vi "Initialize Globals - Engineering.vi"(0 "TSM context":T2, 5 "TCs-Engineering":T1) -> (15 "error out":errorcluster)   [LabVIEW 2019]
uses:
  <vilib>/NI_TestStand_SemiconductorModule/NI_TestStand_Semiconductor_Module.lvlibp/PinMap/General/SemiconductorModuleContext.ctl
  Common/Utility/typedefs/TCs-Engineering.ctl
  TSM Context Data Access/TSM Context Data Access.lvclass/TSM Context Data Access.ctl
  TSM Context Data Access/Public/Properties/TCs-Engineering - Write.vi
  <vilib>/NI_TestStand_SemiconductorModule/NI_TestStand_Semiconductor_Module.lvlibp/PinMap/Site and Global Data/SetGlobalData.vi
  TSM Context Data Access/TSM Context Data Access.lvclass
  <vilib>/NI_TestStand_SemiconductorModule/NI_TestStand_Semiconductor_Module.lvlibp
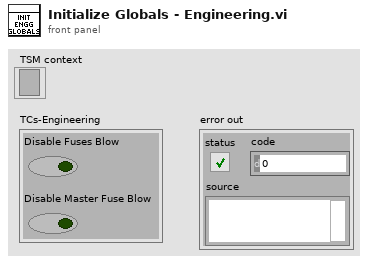
[diagram p1: front panel]
types:
  T1 = typedef "TCs-Engineering.ctl" = cluster{"Disable Fuses Blow":bool, "Disable Master Fuse Blow":bool}
  T2 = typedef "NI_TestStand_Semiconductor_Module.lvlibp/SemiconductorModuleContext.ctl" = refnum<k7>
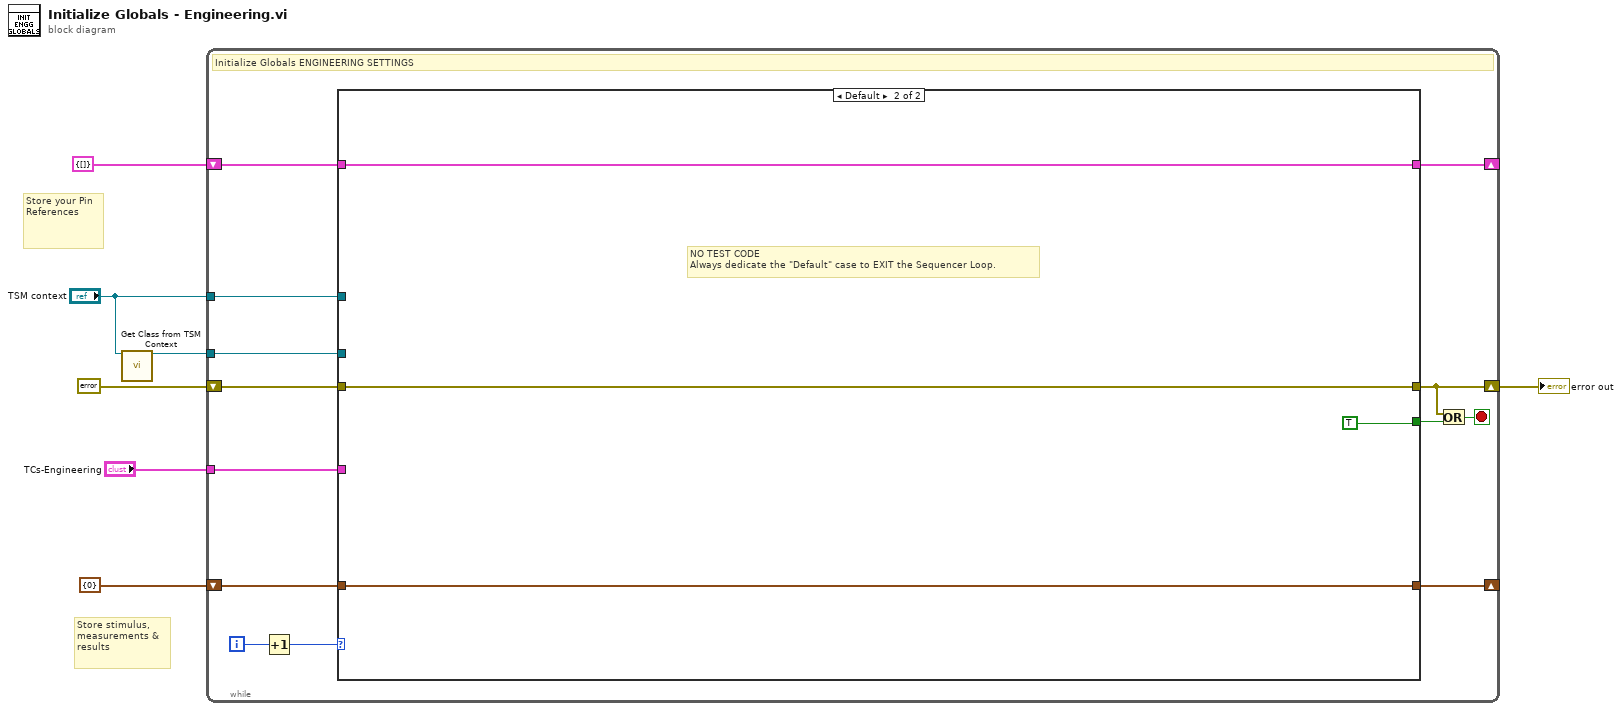
[diagram p0: block diagram]
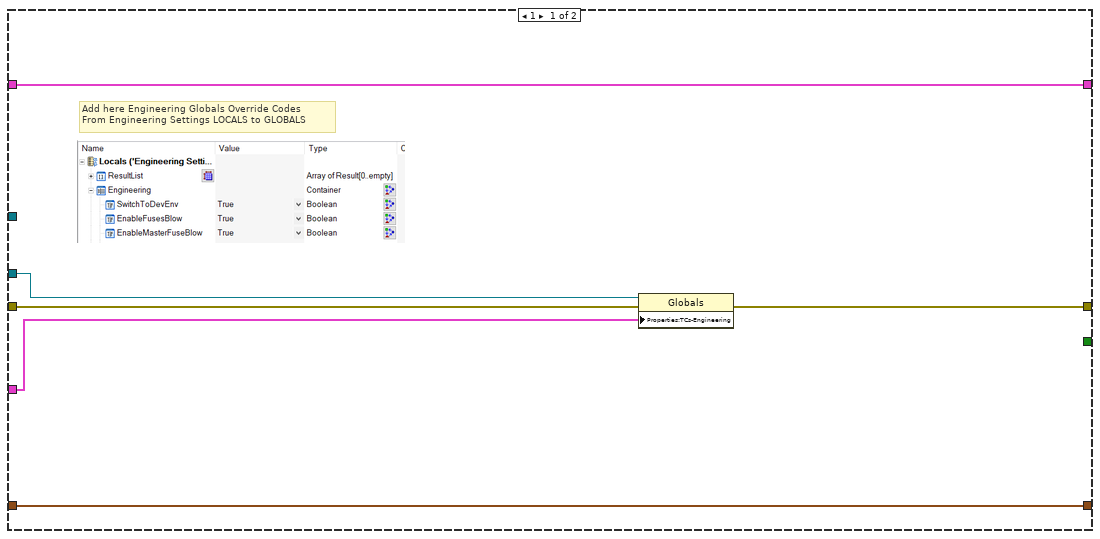
[diagram p2: hidden frame]
diagram:
  # "Store stimulus, measurements & results"
  # "Store your Pin References"
  n1 = call "Get Class from TSM Context.vi"("TSM Context"="TSM context") -> ("Global Memory Class"=w2:refnum<class "TSM Context Data Access.lvclass">)  [unwired: 14 in]
  n2 = while {
    shift-right: [w12] -> w7
    shift-left: errorcluster {"status"=FALSE, "code"=0, "source"=""} ("error in") -> [w19]
    tunnel: "TSM context" -> [w17]
    shift-right: [w14] -> _
    shift-left: cluster{"Site Numbers":i32[]} {"Site Numbers"=[]} -> [w15]
    shift-right: [w11] -> _
    shift-left: cluster{"Sample Control":i32} {"Sample Control"=0} ("TCs") -> [w10]
    tunnel: w2 -> [w9]
    tunnel: "TCs-Engineering" -> [w8]
    i -> [w20]
    stop <- w13 stop-if-true
    # "Initialize Globals ENGINEERING SETTINGS"
    n3 = Increment(x=w20) -> (x+1=w18:i32)
    n4 = case shown="Default" w18 {
      tunnel: [w23 w29] -> w12
      tunnel: w19 -> [w24 w29]
      tunnel: w17 -> [_ _]
      tunnel: [_ TRUE] -> w16
      tunnel: w15 -> [w26 w28]
      tunnel: [w26 w28] -> w14
      tunnel: [w25 w27] -> w11
      tunnel: w10 -> [w25 w27]
      tunnel: w9 -> [w22 _]
      tunnel: w8 -> [w21 _]
      frame 1 {
        # "Add here Engineering Globals Override Codes \nFrom Engineering Settings LOCALS to GLOBALS"
        # "Get Instrument References\nDO NOT CHANGE IF NO ADDITIONAL PINS"
        n5 = property class="Globals"(reference=w22, error in=w24, "Properties:TCs-Engineering"=w21) -> (error out=w23:errorcluster)  [unwired: 1 out]
      }
      frame Default {
        # "NO TEST CODE\nAlways dedicate the \"Default\" case to EXIT the Sequencer Loop."
        # "Exit Loop"
      }
    }
    n6 = Or(x=w12, y=w16) -> (x .or. y?=w13:bool)
  }
  "error out" <- w7
